vi "go_to_wavelength_doubled.vi"(0 "Set Laser Position":dbl, 1 "Set BBO crystal position":i32, 3 "Unit":u16(ring) items=["nm", "cm-1"], 11 "error in (no error)":errorcluster) -> (4 "Current Laser Position":dbl, 15 "error out":errorcluster)   [LabVIEW 2023]
panel:
  out "BBO crystal position":i32
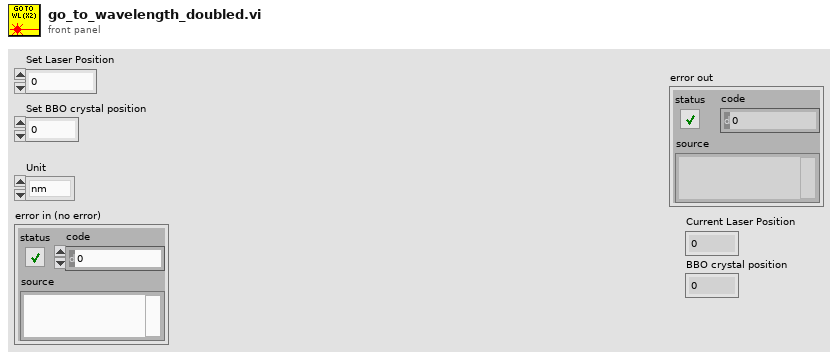
[diagram p1: front panel]
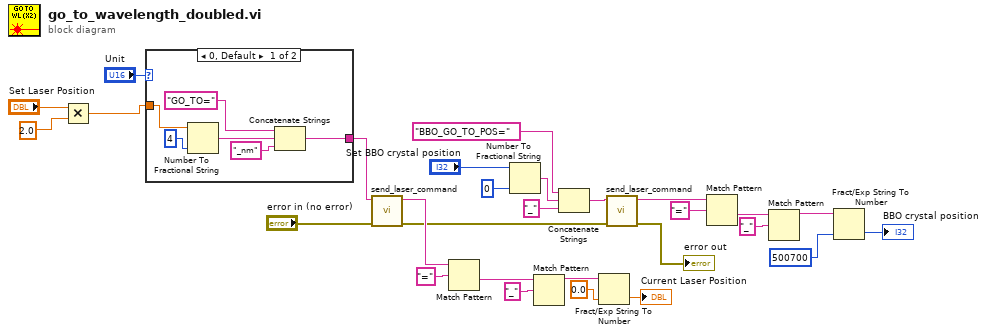
[diagram p0: block diagram]
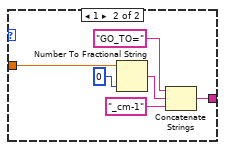
[diagram p2: hidden frame]
diagram:
  n1 = Multiply(x="Set Laser Position", y=2.0) -> (x*y=w2:dbl)
  n2 = case shown="0, Default" "Unit" {
    tunnel: w2 -> [w30 w36]
    tunnel: [w29 w35] -> w28
    frame 0, Default {
      n3 = Number To Fractional String(number=w30, precision (6)=i16 4) -> (F-format string=w32:string)  [unwired: 2 in]
      n4 = Concatenate Strings("GO_TO=", w32, "_nm" ("string")) -> (w29:string)
    }
    frame 1 {
      n5 = Number To Fractional String(number=w36, precision (6)=i16 0) -> (F-format string=w38:string)  [unwired: 2 in]
      n6 = Concatenate Strings("GO_TO=", w38, "_cm-1" ("string")) -> (w35:string)
    }
  }
  n7 = call "send_laser_command.vi"("error in (no error)"="error in (no error)", "String"=w28) -> ("error out"=w5:errorcluster, "data out"=w20:string)  [unwired: 8 in]
  n8 = Match Pattern(string=w20, regular expression="=") -> (after substring=w24:string)  [unwired: 1 in, 3 out]
  n9 = Number To Fractional String(number="Set BBO crystal position", precision (6)=i16 0) -> (F-format string=w11:string)  [unwired: 2 in]
  n10 = Match Pattern(string=w24, regular expression="_") -> (before substring=w22:string)  [unwired: 1 in, 3 out]
  n11 = Concatenate Strings("BBO_GO_TO_POS=", w11, "_" ("string")) -> (w9:string)
  n12 = Fract/Exp String To Number(string=w22, default (0 dbl)=0.0 ("number")) -> (number=→"Current Laser Position":dbl)  [unwired: 2 in, 1 out]
  n13 = call "send_laser_command.vi"("error in (no error)"=w5, "String"=w9) -> ("error out"=→"error out":errorcluster, "data out"=w14:string)  [unwired: 8 in]
  n14 = Match Pattern(string=w14, regular expression="=") -> (after substring=w17:string)  [unwired: 1 in, 3 out]
  n15 = Match Pattern(string=w17, regular expression="_") -> (before substring=w15:string)  [unwired: 1 in, 3 out]
  n16 = Fract/Exp String To Number(string=w15, default (0 dbl)=500700 ("Set BBO crystal position")) -> (number=→"BBO crystal position":i32)  [unwired: 2 in, 1 out]
